vi "Set Text.vi"(8 "Error In":errorcluster, 10 "Text":string, 11 "Pixel In":refnum<class "String.lvclass">) -> (0 "Error Out":errorcluster, 3 "Pixel Out":refnum<class "String.lvclass">)   [LabVIEW 2019, in "String.lvclass"]
uses:
  String.lvclass
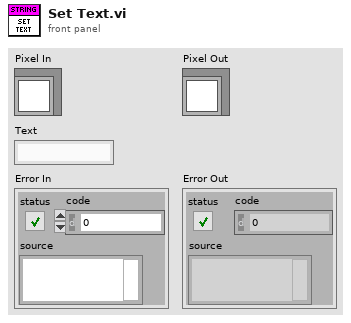
[diagram p1: front panel]
types:
  T1 = typedef "String.lvclass/Data.ctl" = cluster{"Text":string, "Letters Array":void[]}
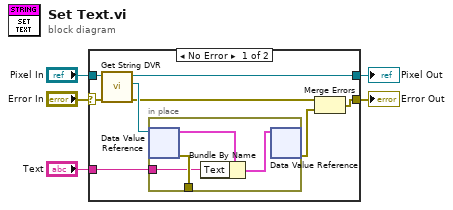
[diagram p0: block diagram]
diagram:
  n1 = case shown="No Error" "Error In" {
    selector: "Error In" -> [w10 w18]
    tunnel: [w12 w18] -> w4
    tunnel: [w7 w19] -> w1
    tunnel: "Pixel In" -> [w9 w19]
    tunnel: "Text" -> [w11 _]
    frame No Error {
      n2 = call "Get String DVR.vi"("Error In"=w10, "Pixel In"=w9) -> ("Error Out"=w6:errorcluster, "DVR"=w8:refnum<data-value>, "Pixel Out"=w7:refnum<class "String.lvclass">)  [unwired: 7 in]
      n3 = in-place {
        in-place-border: [w17] -> _
        in-place-border: w11 -> [w14]
        n4 = in-place-dvr #1(w8) -> (w16:T1, w17:errorcluster)
        n5 = Bundle By Name(cluster=w16, "Text"=w14) -> (w15:T1)
        n6 = in-place-dvr #1(w15) -> (w13:errorcluster)  [unwired: 1 out]
      }
      n7 = Merge Errors(w6, w13) -> (w12:errorcluster)
    }
    frame Error {
    }
  }
  "Pixel Out" <- w1
  "Error Out" <- w4
